vi "Move Right Joints.vi"(5 "Label":string, 6 "Wait (s)":dbl, 8 "error in":errorcluster, 9 "time":dbl=2.0, 10 "Goal":dbl[](array[numeric])) -> (0 "error out":errorcluster)   [LabVIEW 2013]
uses:
  ROS/Code/Console/Servers/ServerSubs/(nist) Arm Globals.vi
panel:
  # "All Joint motions\nare relative to BASE"
  # "Cannot make\njoint motions \nvertical"
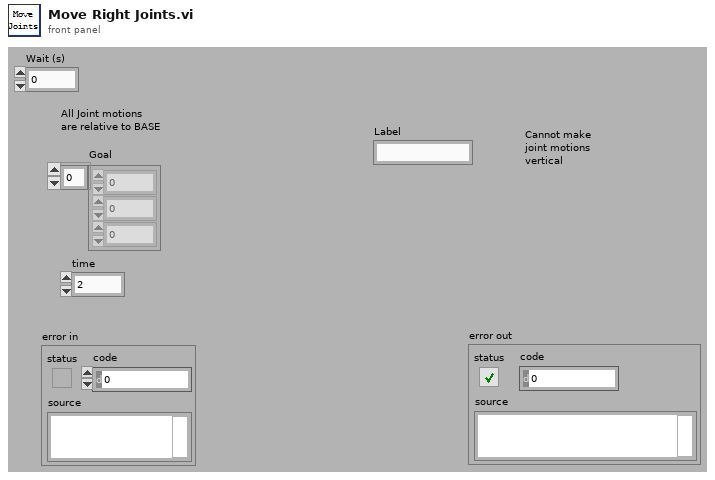
[diagram p1: front panel]
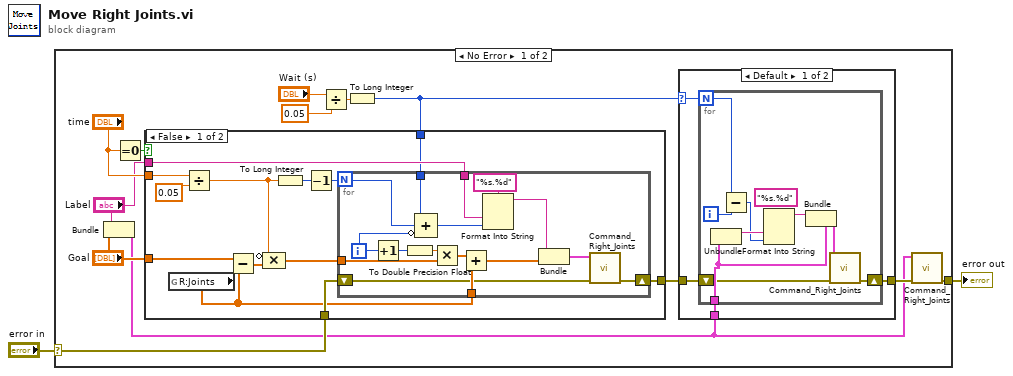
[diagram p0: block diagram]
diagram:
  n1 = case shown="No Error" "error in" {
    selector: "error in" -> [w6 w60]
    tunnel: [w4 w60] -> w1
    frame No Error {
      n2 = Bundle("Label"="Label", "Goal"="Goal") -> (w3:cluster{"Label":string, "Goal":dbl[]})  [unwired: 1 in]
      n3 = Equal To 0?(x="time") -> (x = 0?=w15:bool)
      n4 = Divide(x="Wait (s)", y=0.05) -> (x/y=w9:dbl)
      n5 = To Long Integer(number=w9) -> (32bit integer=w8:i32)
      n6 = case shown="False" w15 {
        tunnel: "Label" -> [w39 _]
        tunnel: "Goal" -> [w33 _]
        tunnel: "time" -> [w42 _]
        tunnel: w8 -> [w34 _]
        tunnel: [w31 w59] -> w7
        tunnel: w6 -> [w32 w59]
        frame False {
          n7 = global read "(nist) Arm Globals.vi" "R:Joints"() -> (w30:dbl[])
          n8 = Divide(x=w42, y=0.05) -> (x/y=w35:dbl)
          n9 = Subtract(x=w33, y=w30) -> (x-y=w36:dbl[])
          n10 = Compound Arithmetic op=MULTIPLY(invert w35, w36) -> (w37:dbl[])
          n11 = To Long Integer(number=w35) -> (32bit integer=w40:i32)
          n12 = Decrement(x=w40) -> (x-1=w38:i32)
          n13 = for {
            N: w38 -> [w58]
            tunnel: w37 -> [w55]
            tunnel: w39 -> [w53]
            tunnel: w34 -> [w50]
            tunnel: w30 -> [w48]
            shift-right: [w46] -> w31
            shift-left: w32 -> [w47]
            i -> [w57]
            n14 = Increment(x=w57) -> (x+1=w51:i32)
            n15 = To Double Precision Float(number=w51) -> (double precision float=w56:dbl)
            n16 = Compound Arithmetic op=ADD(w50, w58, invert w57) -> (w52:i32)
            n17 = Multiply(x=w56, y=w55) -> (x*y=w49:dbl[])
            n18 = Add(x=w49, y=w48) -> (x+y=w44:dbl[])
            n19 = Format Into String(format string="%s.%d", w53, w52) -> (resulting string=w45:string)  [unwired: 2 in, 1 out]
            n20 = Bundle(w45, w44) -> (w43:cluster{string, dbl[]})  [unwired: 1 in]
            n21 = call "Command_Right_Joints.vi"("error in"=w47, "Goal"=w43) -> ("error out"=w46:errorcluster)  [unwired: 6 in, 1 out]
          }
        }
        frame True {
        }
      }
      n22 = case shown="Default" w8 {
        selector: w8 -> [w16 _]
        tunnel: w7 -> [w19 w29]
        tunnel: [w18 w29] -> w5
        tunnel: w3 -> [w17 _]
        frame Default {
          n23 = for {
            N: w16 -> [w28]
            tunnel: w17 -> [w23]
            shift-right: [w21] -> w18
            shift-left: w19 -> [w22]
            i -> [w27]
            (unwired) "%s.%d" ("format string")
            n24 = Unbundle(w23) -> ("Label"=w26:string)  [unwired: 1 out]
            n25 = Subtract(x=w28, y=w27) -> (x-y=w25:i32)
            n26 = Format Into String(w26, w25) -> (resulting string=w24:string)  [unwired: 3 in, 1 out]
            n27 = Bundle(cluster=w23, "Label"=w24) -> (w20:cluster{"Label":string, "Goal":dbl[]})  [unwired: 1 in]
            n28 = call "Command_Right_Joints.vi"("error in"=w22, "Goal"=w20) -> ("error out"=w21:errorcluster)  [unwired: 6 in, 1 out]
          }
        }
        frame 0 {
        }
      }
      n29 = call "Command_Right_Joints.vi"("error in"=w5, "Goal"=w3) -> ("error out"=w4:errorcluster)  [unwired: 6 in, 1 out]
    }
    frame Error {
    }
  }
  "error out" <- w1
